vi "Move Slot.vi"(8 "error in":errorcluster, 10 "destination slot ref in":T1 format="%.0x", 11 "source slot ref in":T1 format="%.0x") -> (0 "error out":errorcluster, 2 "destination slot ref out":T1 format="%.0x", 3 "source slot ref out":T1 format="%.0x")   [LabVIEW 2017, in "Scan Engine Scripting.lvlib"]
uses:
  Scan Engine Scripting.lvlib
  <vilib>/NI Veristand/Custom Device API/Custom Device Item Ref.ctl
  <vilib>/NI Veristand/Custom Device API/Custom Device API.lvlib
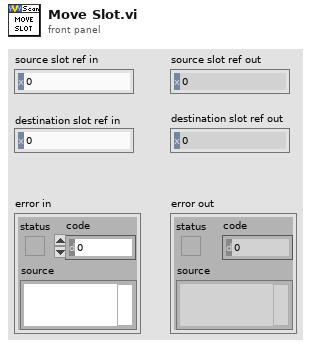
[diagram p1: front panel]
types:
  T1 = typedef "Custom Device API.lvlib/Custom Device Item Ref.ctl" = u64
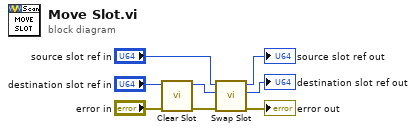
[diagram p0: block diagram]
diagram:
  n1 = call "Clear Slot.vi"("error in"="error in", "slot ref in"="destination slot ref in") -> ("error out"=w7:errorcluster, "slot ref out"=w4:T1)  [unwired: 8 in]
  n2 = call "Swap Slot.vi"("error in"=w7, "slot 2 ref in"=w4, "slot 1 ref in"="source slot ref in") -> ("error out"=→"error out":errorcluster, "slot 2 ref out"=→"destination slot ref out":T1, "slot 1 ref out"=→"source slot ref out":T1)  [unwired: 6 in]
